vi "Serialize - JSON.vi"(8 "error in (no error)":errorcluster, 11 "ePAS Cell Data in":refnum<class "ePAS Cell Data.lvclass">) -> (0 "error out":errorcluster, 2 "Serialized JSON":string, 3 "ePAS Cell Data out":refnum<class "ePAS Cell Data.lvclass">)   [LabVIEW 2014, in "ePAS Library.lvlib" / "ePAS Cell Data.lvclass"]
uses:
  ePAS Cell Data.lvclass
  ePAS Cell Data.lvclass/ePAS Cell Data.ctl
  reusable/PAS/Data/Cell/PAS Cell Data.lvclass
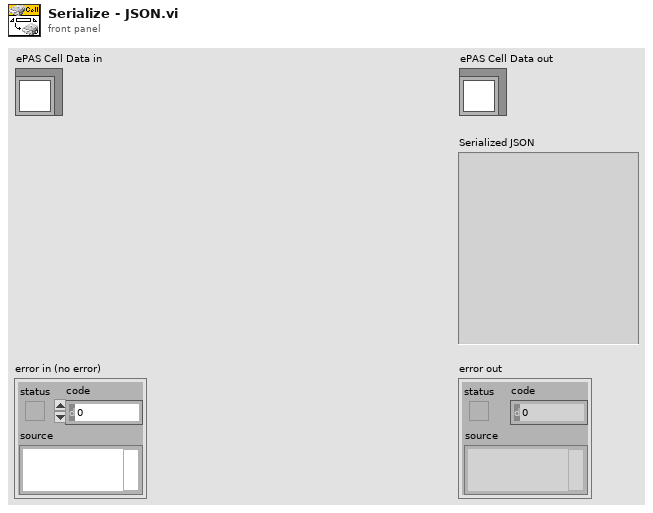
[diagram p1: front panel]
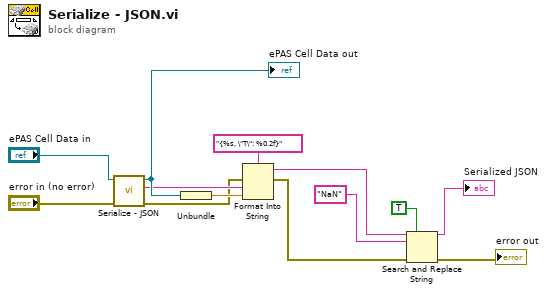
[diagram p0: block diagram]
diagram:
  n1 = call-parent "Serialize - JSON.vi"("error in"="error in (no error)", "PAS Cell Data in"="ePAS Cell Data in") -> ("error out"=w3:errorcluster, "Serialized JSON"=w5:string, "PAS Cell Data out"=w11:refnum<class "ePAS Cell Data.lvclass">)  [unwired: 7 in]
  "ePAS Cell Data out" <- w11
  n2 = Unbundle(w11) -> (w6:dbl)
  n3 = Format Into String(format string="{%s, \"T\": %0.2f}", error in=w3, w5, w6) -> (resulting string=w4:string, error out=w2:errorcluster)  [unwired: 1 in]
  n4 = Search and Replace String(replace all?=TRUE ("replace all? (F)"), input string=w4, search string="NaN", error in=w2) -> (result string=→"Serialized JSON":string, error out=→"error out":errorcluster)  [unwired: 4 in, 2 out]
